vi "ctx restore context from disk.vi"(10 "filepath":string, 11 "context":u32) -> (2 "function return":i32, 3 "context out":u32)   [LabVIEW 2019, in "apdm.lvlib"]
doc: "APDM_EXPORT int apdm_ctx_restore_context_from_disk(apdm_ctx_t context, const char *filepath);"
uses:
  apdm.lvlib
  Lee Lab/CP FES Walking 2018/Code/Working/LabVIEW/apdm.dll
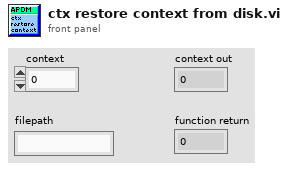
[diagram p1: front panel]
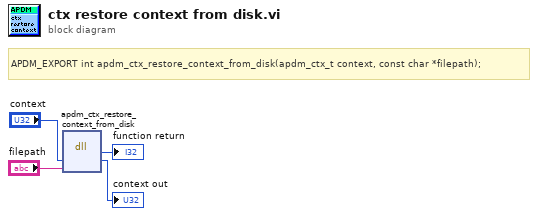
[diagram p0: block diagram]
diagram:
  # "APDM_EXPORT int apdm_ctx_restore_context_from_disk(apdm_ctx_t context, const char *filepath);"
  n1 = dll-call lib="C:/Users/jfalesi/Dropbox/Lee Lab/CP FES Walking 2018/Code/Working/LabVIEW/apdm.*" fn="apdm_ctx_restore_context_from_disk"("context"="context", "filepath"="filepath") -> (→"function return":i32, "context"=→"context out":u32)  [unwired: 4 in, 2 out]
